vi "Define connected systems.vi"(0 "System no.":i32=1 min=1 max=4 step=1, 3 "Change only one system?":bool, 4 "Controller names":T2, 5 "error in":errorcluster) -> (14 "Controller names out":T2, 19 "error out":errorcluster)   [LabVIEW 2020]
doc: "Defines connected systems and writes controller names into Global2.vi. This VI is called automatically by PI_GCS2_Configuration_Setup.vi and must be completed successfully before General wait for movement to stop.vi is called. If Change only one system? is FALSE, all four entries from Controller names are written into Global2.vi. If Change only one system? is TRUE, only the entry for the given system number is overwritten in Global2.vi.\nOld VI - only for compatibility reasons available. Limited to 4 systems. Use Define connected systems (Array).vi instead."
uses:
  General command.llb/Controller names.ctl
  General command.llb/Global2 (Array).vi
panel:
  # "Defines connected systems and writes controller names into Global2.vi.\nIf \"Change only one system?\" is FALSE, all four entries from \"Controller\nnames\" are written into Global2.vi. If \"Change only one system?\" is TRUE,\nonly the entry for the given system number is overwritten in Global2.vi.\nOld VI - only for compatibility reasons available. Limited to 4 systems. \nUse Define connected systems (Array).vi instead."
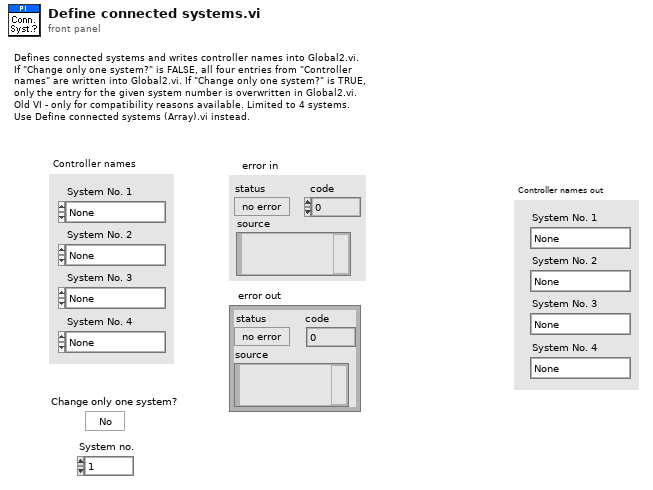
[diagram p1: front panel]
types:
  T1 = typedef "Controller names.ctl" = enum16{"None", "Analog", "C-702", "C-413", "C-414", "C-843", "C-843.PM", "C-844", "C-848", "C-865", "C-866", "C-867", "C-877", "C-880", "C-884", "C-885", "C-886", "C-887", "C-891", "E-135", "E-516", "E-517", "E-518", "E-709", "E-710", "E-712", "E-725", "E-727", "E-753", "E-754", "E-755", "E-761", "E-816", "E-861", "E-870", "E-871", "E-872", "E-873", "E-874", "F-206", "HydraPollux", "M-840", "M-850", "M-8X0", "Mercury", "Mercury_GCS", "PI_GCS2"}
  T2 = cluster{"System No. 1":T1, "System No. 2":T1, "System No. 3":T1, "System No. 4":T1}
  T3 = cluster{"System No. 1":enum16{"None", "C-843", "C-844", "C-848", "C-880", "E-516", "E-816", "F-206", "M-840", "M-850"}, "System No. 2":enum16{"None", "C-843", "C-844", "C-848", "C-880", "E-516", "E-816", "F-206", "M-840", "M-850"}, "System No. 3":enum16{"None", "C-843", "C-844", "C-848", "C-880", "E-516", "E-816", "F-206", "M-840", "M-850"}, "System No. 4":enum16{"None", "C-843", "C-844", "C-848", "C-880", "E-516", "E-816", "F-206", "M-840", "M-850"}}
  T4 = cluster{"Conn. axes":string[], "Controller name":T1}[]
  T5 = cluster{"Conn. axes":string[], "Controller name":T1}
  T6 = cluster{"Controller name":T1, "Controller name":T1, "Controller name":T1, "Controller name":T1}
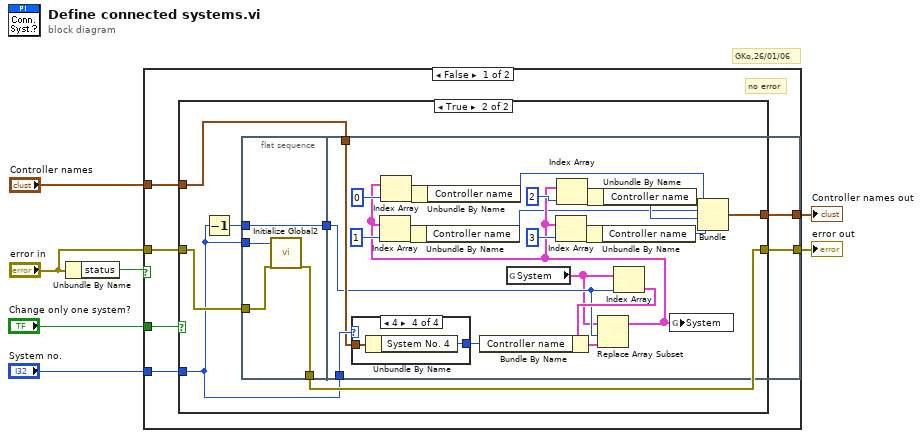
[diagram p0: block diagram]
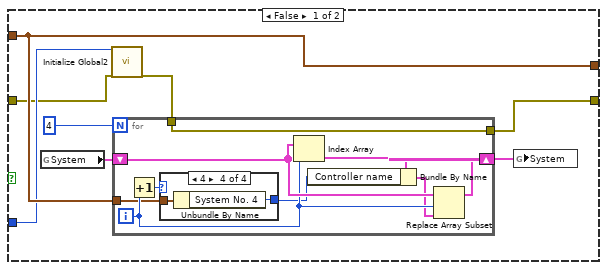
[diagram p2: hidden frame]
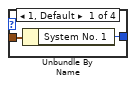
[diagram p3: hidden frame]
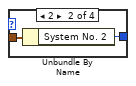
[diagram p4: hidden frame]
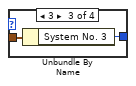
[diagram p5: hidden frame]
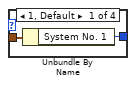
[diagram p6: hidden frame]
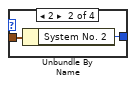
[diagram p7: hidden frame]
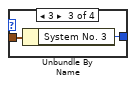
[diagram p8: hidden frame]
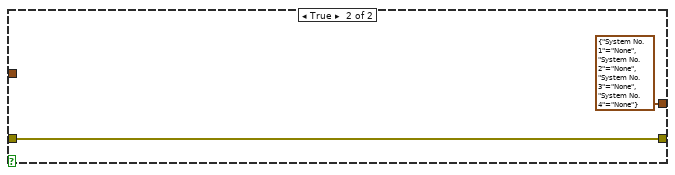
[diagram p9: hidden frame]
diagram:
  # "GKo,26/01/06"
  n1 = Unbundle By Name("error in") -> ("status"=w6:bool)
  n2 = case shown="False" w6 {
    tunnel: "Controller names" -> [w13 _]
    tunnel: "error in" -> [w11 w80]
    tunnel: [w10 w80] -> w4
    tunnel: "Change only one system?" -> [w12 _]
    tunnel: "System no." -> [w9 _]
    tunnel: [w8 T3 {"System No. 1"=enum."None", "System No. 2"=enum."None", "System No. 3"=enum."None", "System No. 4"=enum."None"} ("Controller names")] -> w1
    frame False {
      # "no error"
      n3 = case shown="True" w12 {
        tunnel: w13 -> [w18 w41]
        tunnel: w11 -> [w16 w44]
        tunnel: [w14 w43] -> w10
        tunnel: w9 -> [w17 w39]
        tunnel: [w18 w40] -> w8
        frame False {
          n4 = global read "Global2 (Array).vi" "System"() -> (w20:T4)
          n5 = call "Initialize Global2.vi"("System no."=w17, "error in"=w16) -> ("error out"=w15:errorcluster)  [unwired: 17 out]
          n6 = for {
            N: 4 -> [_]
            shift-right: [w26] -> w19
            shift-left: w20 -> [w30]
            tunnel: w18 -> [w27]
            tunnel: [w22] -> w14
            tunnel: w15 -> [w22]
            i -> [w29]
            n7 = Increment(x=w29) -> (x+1=w28:i32)
            n8 = case shown="4" w28 {
              tunnel: w27 -> [w32 w34 w36 w38]
              tunnel: [w31 w33 w35 w37] -> w24
              frame 1, Default {
                n9 = Unbundle By Name(w32) -> ("System No. 1"=w31:T1)
              }
              frame 2 {
                n10 = Unbundle By Name(w34) -> ("System No. 2"=w33:T1)
              }
              frame 3 {
                n11 = Unbundle By Name(w36) -> ("System No. 3"=w35:T1)
              }
              frame 4 {
                n12 = Unbundle By Name(w38) -> ("System No. 4"=w37:T1)
              }
            }
            n13 = Index Array(array=w30, index=w29) -> (element=w25:T5)
            n14 = Bundle By Name(cluster=w25, "Controller name"=w24) -> (w23:T5)
            n15 = Replace Array Subset(array=w30, new element=w23, index=w29) -> (w26:T4)
          }
          n16 = global write "Global2 (Array).vi" "System"(w19) -> ()
        }
        frame True {
          n17 = Decrement(x=w39) -> (x-1=w45:i32)
          n18 = flat-sequence {
            tunnel: w45 -> [w47]
            tunnel: w44 -> [w49]
            tunnel: [w48] -> w43
            tunnel: [w47] -> w42
            tunnel: w39 -> [w46]
            tunnel: w39 -> [w70]
            tunnel: w42 -> [w65]
            tunnel: w41 -> [w69]
            tunnel: [w51] -> w40
            frame #0 {
              n19 = call "Initialize Global2.vi"("System no."=w46, "error in"=w49) -> ("error out"=w48:errorcluster)  [unwired: 17 out]
            }
            frame #1 {
              n20 = case shown="4" w70 {
                tunnel: w69 -> [w72 w74 w76 w78]
                tunnel: [w71 w73 w75 w77] -> w67
                frame 1, Default {
                  n21 = Unbundle By Name(w72) -> ("System No. 1"=w71:T1)
                }
                frame 2 {
                  n22 = Unbundle By Name(w74) -> ("System No. 2"=w73:T1)
                }
                frame 3 {
                  n23 = Unbundle By Name(w76) -> ("System No. 3"=w75:T1)
                }
                frame 4 {
                  n24 = Unbundle By Name(w78) -> ("System No. 4"=w77:T1)
                }
              }
              n25 = global read "Global2 (Array).vi" "System"() -> (w50:T4)
              n26 = Index Array(array=w50, index=w65) -> (element=w68:T5)
              n27 = Bundle By Name(cluster=w68, "Controller name"=w67) -> (w66:T5)
              n28 = Replace Array Subset(array=w50, new element=w66, index=w65) -> (w56:T4)
              n29 = Index Array(array=w56, index=1) -> (element=w60:T5)
              n30 = Index Array(array=w56, index=0) -> (element=w64:T5)
              n31 = Unbundle By Name(w60) -> ("Controller name"=w53:T1)
              n32 = Unbundle By Name(w64) -> ("Controller name"=w52:T1)
              n33 = Index Array(array=w56, index=3) -> (element=w58:T5)
              n34 = Index Array(array=w56, index=2) -> (element=w62:T5)
              n35 = Unbundle By Name(w58) -> ("Controller name"=w55:T1)
              n36 = Unbundle By Name(w62) -> ("Controller name"=w54:T1)
              n37 = global write "Global2 (Array).vi" "System"(w56) -> ()
              n38 = Bundle("Controller name"=w52, "Controller name"=w53, "Controller name"=w54, "Controller name"=w55) -> (w51:T6)  [unwired: 1 out]
            }
          }
        }
      }
    }
    frame True {
    }
  }
  "error out" <- w4
  "Controller names out" <- w1
